vi "FGV Timer.vi"(8 "Error In":errorcluster, 9 "Timer Option":T1, 10 "Target Time":dbl) -> (0 "Error Out":errorcluster, 1 "Timer Has Elapsed?":bool, 2 "Time Elapsed":dbl)   [LabVIEW 2015]
doc: "This FGV VI is used to create a Timer that has function of Start, Read and Pause."
uses:
  controls/Timer Option.ctl
panel:
  # "FGV TIMER VI"
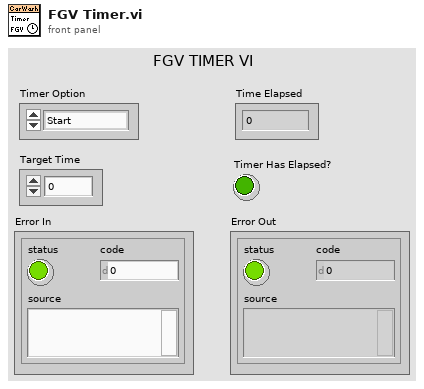
[diagram p1: front panel]
types:
  T1 = typedef "Timer Option.ctl" = enum16{"Start", "Read", "Pause"}
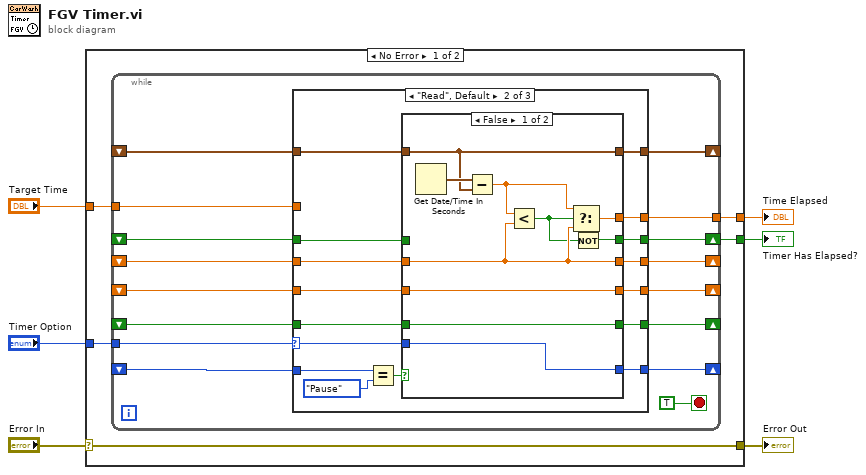
[diagram p0: block diagram]
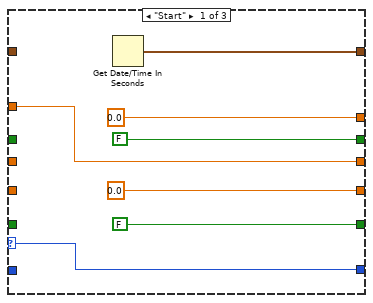
[diagram p2: hidden frame]
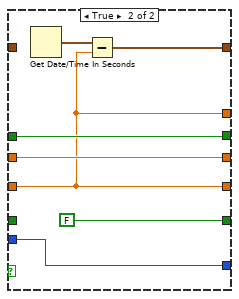
[diagram p3: hidden frame]
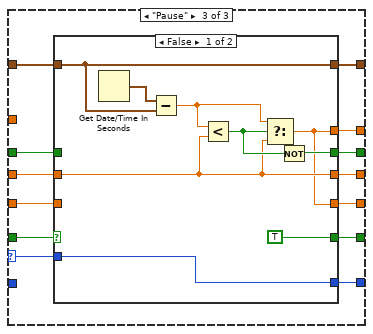
[diagram p4: hidden frame]
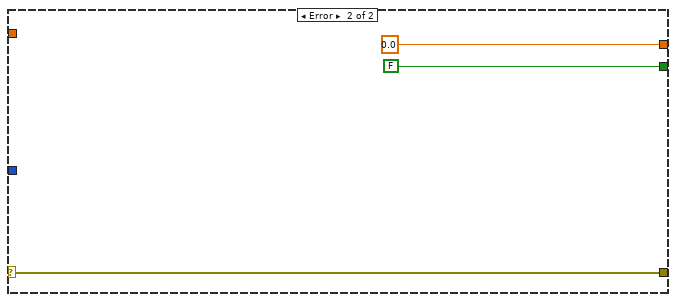
[diagram p6: hidden frame]
diagram:
  n1 = case shown="No Error" "Error In" {
    selector: "Error In" -> [w10 w98]
    tunnel: "Timer Option" -> [w11 _]
    tunnel: [w10 w98] -> w4
    tunnel: "Target Time" -> [w9 _]
    tunnel: [w8 0.0 ("Target Time")] -> w2
    tunnel: [w7 FALSE] -> w1
    frame No Error {
      n2 = while {
        tunnel: w11 -> [w26]
        tunnel: w9 -> [w25]
        shift-right: [w24] -> _
        shift-left: _ -> [w23]
        shift-right: [w22] -> _
        shift-left: _ -> [w21]
        shift-right: [w20] -> _
        shift-left: _ -> [w19]
        tunnel: [w18] -> w8
        shift-right: [w15] -> _
        shift-left: _ -> [w16]
        shift-right: [w17] -> w7
        shift-left: _ -> [w14]
        shift-right: [w13] -> _
        shift-left: _ -> [w12]
        stop <- TRUE stop-if-true
        n3 = case shown="\"Read\", Default" w26 {
          selector: w26 -> [w32 w41 w74]
          tunnel: w25 -> [w34 _ _]
          tunnel: [w34 w45 w78] -> w24
          tunnel: w23 -> [_ w44 w77]
          tunnel: [w33 w50 w80] -> w22
          tunnel: w21 -> [_ w49 w79]
          tunnel: [w32 w40 w73] -> w20
          tunnel: w19 -> [_ w46 _]
          tunnel: [0.0 w43 w76] -> w18
          tunnel: [FALSE w42 w75] -> w17
          tunnel: w16 -> [_ w36 w72]
          tunnel: [FALSE w37 w71] -> w15
          tunnel: w14 -> [_ w38 w70]
          tunnel: [0.0 ("Target Time") w35 w69] -> w13
          tunnel: w12 -> [_ w39 w68]
          frame "Start" {
            n4 = Get Date/Time In Seconds() -> (seconds since 1Jan1904=w33:timestamp)
          }
          frame "Read", Default {
            n5 = Equal?(x=w46, y=Timer_Option."Pause" ("Timer Option")) -> (x = y?=w48:bool)
            n6 = case shown="False" w48 {
              tunnel: w49 -> [w59 _]
              tunnel: [w59 w64] -> w50
              tunnel: [w56 w66] -> w45
              tunnel: w44 -> [w56 w66]
              tunnel: [w57 w61] -> w43
              tunnel: [w54 w63] -> w42
              tunnel: w41 -> [w53 w65]
              tunnel: [w53 w65] -> w40
              tunnel: w39 -> [w51 w61]
              tunnel: w38 -> [_ w63]
              tunnel: [w52 FALSE] -> w37
              tunnel: w36 -> [w52 _]
              tunnel: [w51 w61] -> w35
              frame False {
                n7 = Get Date/Time In Seconds() -> (seconds since 1Jan1904=w60:timestamp)
                n8 = Subtract(x=w60, y=w59) -> (x-y=w58:dbl)
                n9 = Less?(x=w58, y=w56) -> (x < y?=w55:bool)
                n10 = Select(t=w58, s=w55, f=w56) -> (s? t:f=w57:dbl)
                n11 = Not(x=w55) -> (.not. x?=w54:bool)
              }
              frame True {
                n12 = Get Date/Time In Seconds() -> (seconds since 1Jan1904=w67:timestamp)
                n13 = Subtract(x=w67, y=w61) -> (x-y=w64:timestamp)
              }
            }
          }
          frame "Pause" {
            n14 = case shown="False" w72 {
              selector: w72 -> [_ w95]
              tunnel: w79 -> [w85 w90]
              tunnel: [w81 w91] -> w76
              tunnel: w77 -> [w84 w92]
              tunnel: [w86 w93] -> w75
              tunnel: [w85 w90] -> w80
              tunnel: [w84 w92] -> w78
              tunnel: w74 -> [w83 w94]
              tunnel: [w83 w94] -> w73
              tunnel: [TRUE w95] -> w71
              tunnel: w70 -> [_ w93]
              tunnel: [w81 w91] -> w69
              tunnel: w68 -> [_ w91]
              frame False {
                n15 = Get Date/Time In Seconds() -> (seconds since 1Jan1904=w89:timestamp)
                n16 = Subtract(x=w89, y=w85) -> (x-y=w88:dbl)
                n17 = Less?(x=w88, y=w84) -> (x < y?=w87:bool)
                n18 = Select(t=w88, s=w87, f=w84) -> (s? t:f=w81:dbl)
                n19 = Not(x=w87) -> (.not. x?=w86:bool)
              }
              frame True {
              }
            }
          }
        }
      }
    }
    frame Error {
    }
  }
  "Error Out" <- w4
  "Time Elapsed" <- w2
  "Timer Has Elapsed?" <- w1
